vi "HoppingStepModified(XYWithin_And_Nonlinear).vi"() -> ()   [LabVIEW 2014]
uses:
  <vilib>/Platform/TimedLoop/XDataNode/timing_clust.ctl
  <vilib>/Platform/TimedLoop/XDataNode/nitl_modes.ctl
  <vilib>/Platform/TimedLoop/XDataNode/wakeup.ctl
  <vilib>/rvi/Emulation/niFpgaSctlEmulationGetInTimedLoop.vi
  <vilib>/rvi/Emulation/niFpgaProcessEmulError.vi
  <vilib>/rvi/Emulation/niFpgaGetClockAttributes.vi
  <vilib>/rvi/Emulation/niFpgaEmulationReportErrorSimple.vi
  <vilib>/rvi/eio/common/nirviEmuTemplateMethod_errors.vi
  <vilib>/rvi/Emulation/niFpgaCriticalErrorInLSC.vi
  <vilib>/rvi/interface/RandomDataEmulation/niFpgaRandomDataHandleErrors.vi
  <vilib>/eio/EIONode/EIONode.xnode
  <vilib>/Platform/TimedLoop/XDataNode/XDataNode.xnode
  <vilib>/rvi/DataTransferAndStorage/Container/XNode/niFpgaContainer.xnode
  <vilib>/rvi/interface/RandomDataEmulation/nirviRandomDataFpgaReadWriteTemplate.vi
  <vilib>/Platform/TimedLoop/XDataNode/XDNodeRunTimeDep.lvlib
panel:
  out "x >= y?":bool
  out "x*y":i32
  out "CurrDeclineR":i16
  out "ZFreshPos":i16(graph)
  out "Time":i32(graph)
  out "Len":i16(graph)
  out "ZPresPos":i16(graph)
  out "Waveform Chart":i16(graph)
  in  "stop":bool
  in  "MajorWithdraw":i16
  in  "ZOffset":i16
  in  "XNum":i16
  in  "XStepIndex":i16
  in  "XOffset":i16
  in  "YNum":i16
  in  "YStepIndex":i16
  in  "YOffset":i16
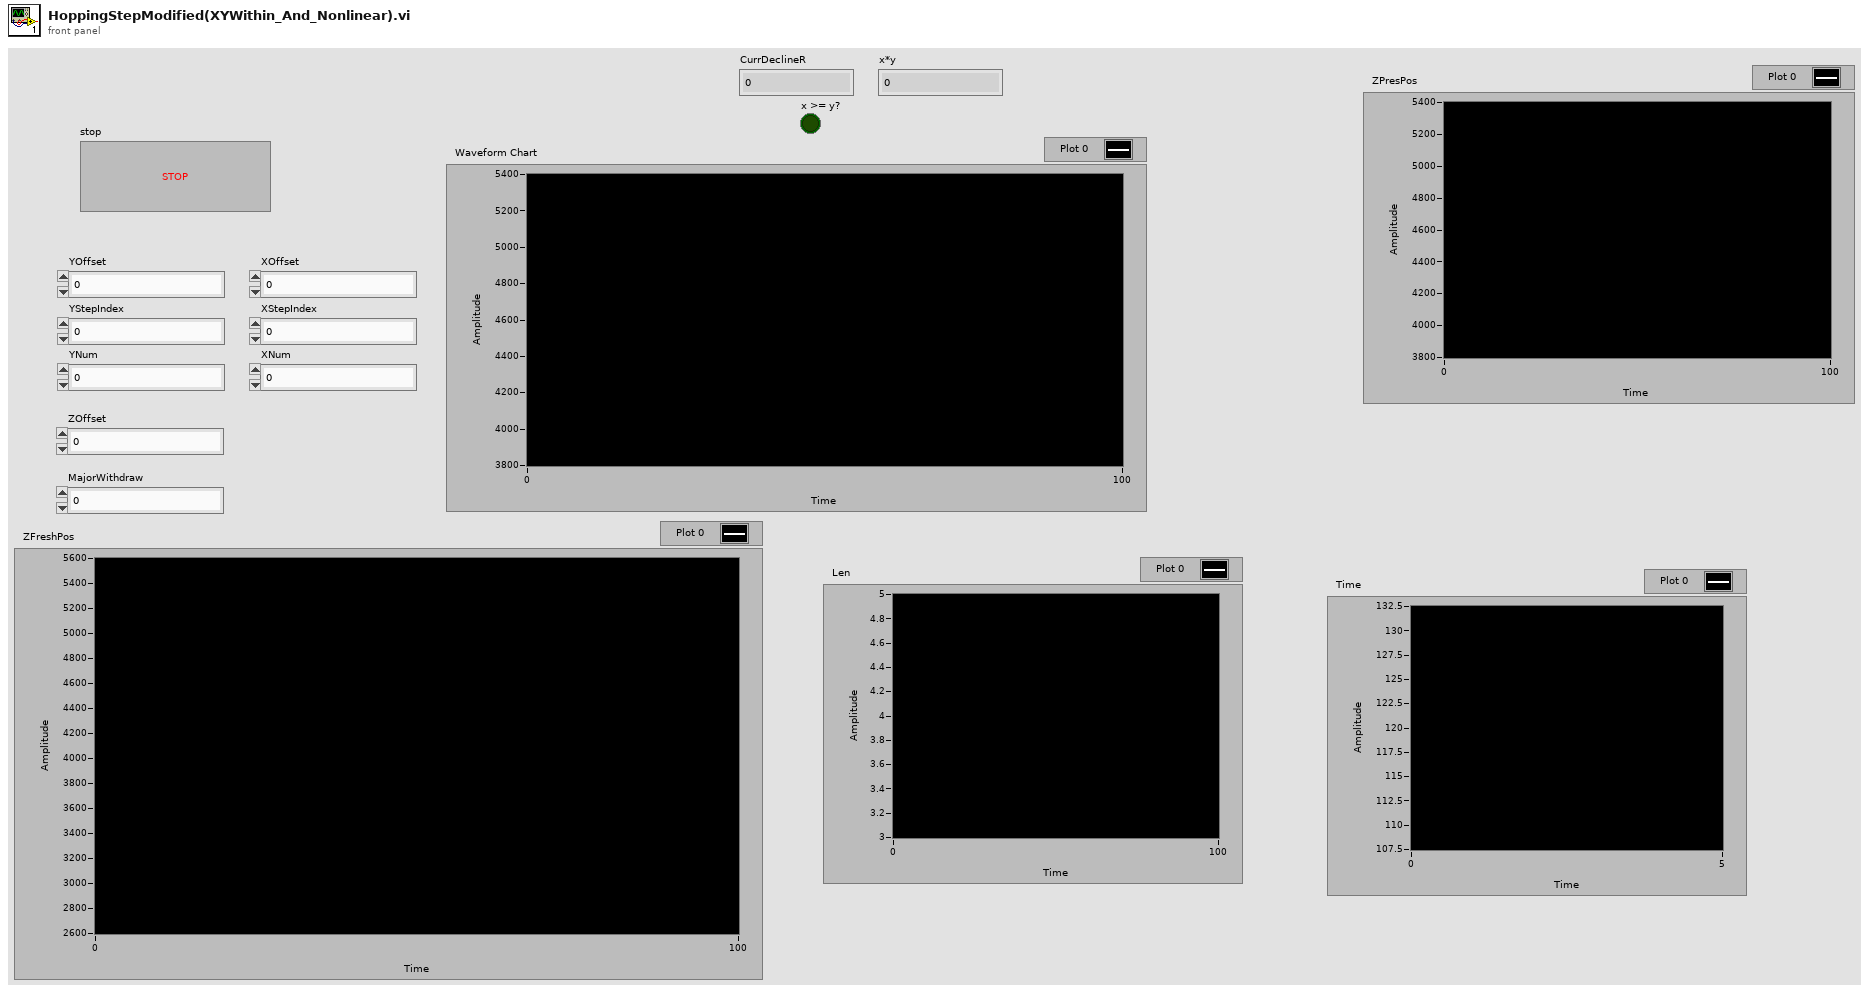
[diagram p1: front panel]
types:
  T1 = typedef "XDNodeRunTimeDep.lvlib/timing_clust.ctl" = cluster{"Expected End [f-1]":u64, "Actual End [f-1]":u64, "Finished Late? [f-1]":bool, "Expected End [i-1]":u64, "Actual End [i-1]":u64, "Finished Late? [i-1]":bool, "Expected Start [i]":u64, "Actual Start [i]":u64, "Expected Start [f]":u64, "Actual Start [f]":u64, "Source Name":string, "Structure Name":string, "Period":i64, "Deadline":i64, "Offset":i64, "Start":i64, "Priority":i32, "Timeout":i32, "Mode":T2, "Wakeup Reason":T3, "Error":errorcluster, "Source Type":string, "Secondary Source Type":string, "Global End Time":u64, "Global Start Time":u64, "Frame Duration":u64, "Iteration Duration":u64, "Assigned CPU":i32, "I/O Scan Engine Mode":u32}
  T2 = typedef "XDNodeRunTimeDep.lvlib/nitl_modes.ctl" = enum32{"No Change", "Process missed periods, maintain original phase", "Discard missed periods, maintain original phase", "Process missed periods, ignore original phase", "Discard missed periods, ignore original phase"}
  T3 = typedef "XDNodeRunTimeDep.lvlib/wakeup.ctl" = enum32{"Normal", "Aborted", "Asynchronous wakeup", "Timing source error", "Timed loop error", "Timeout"}
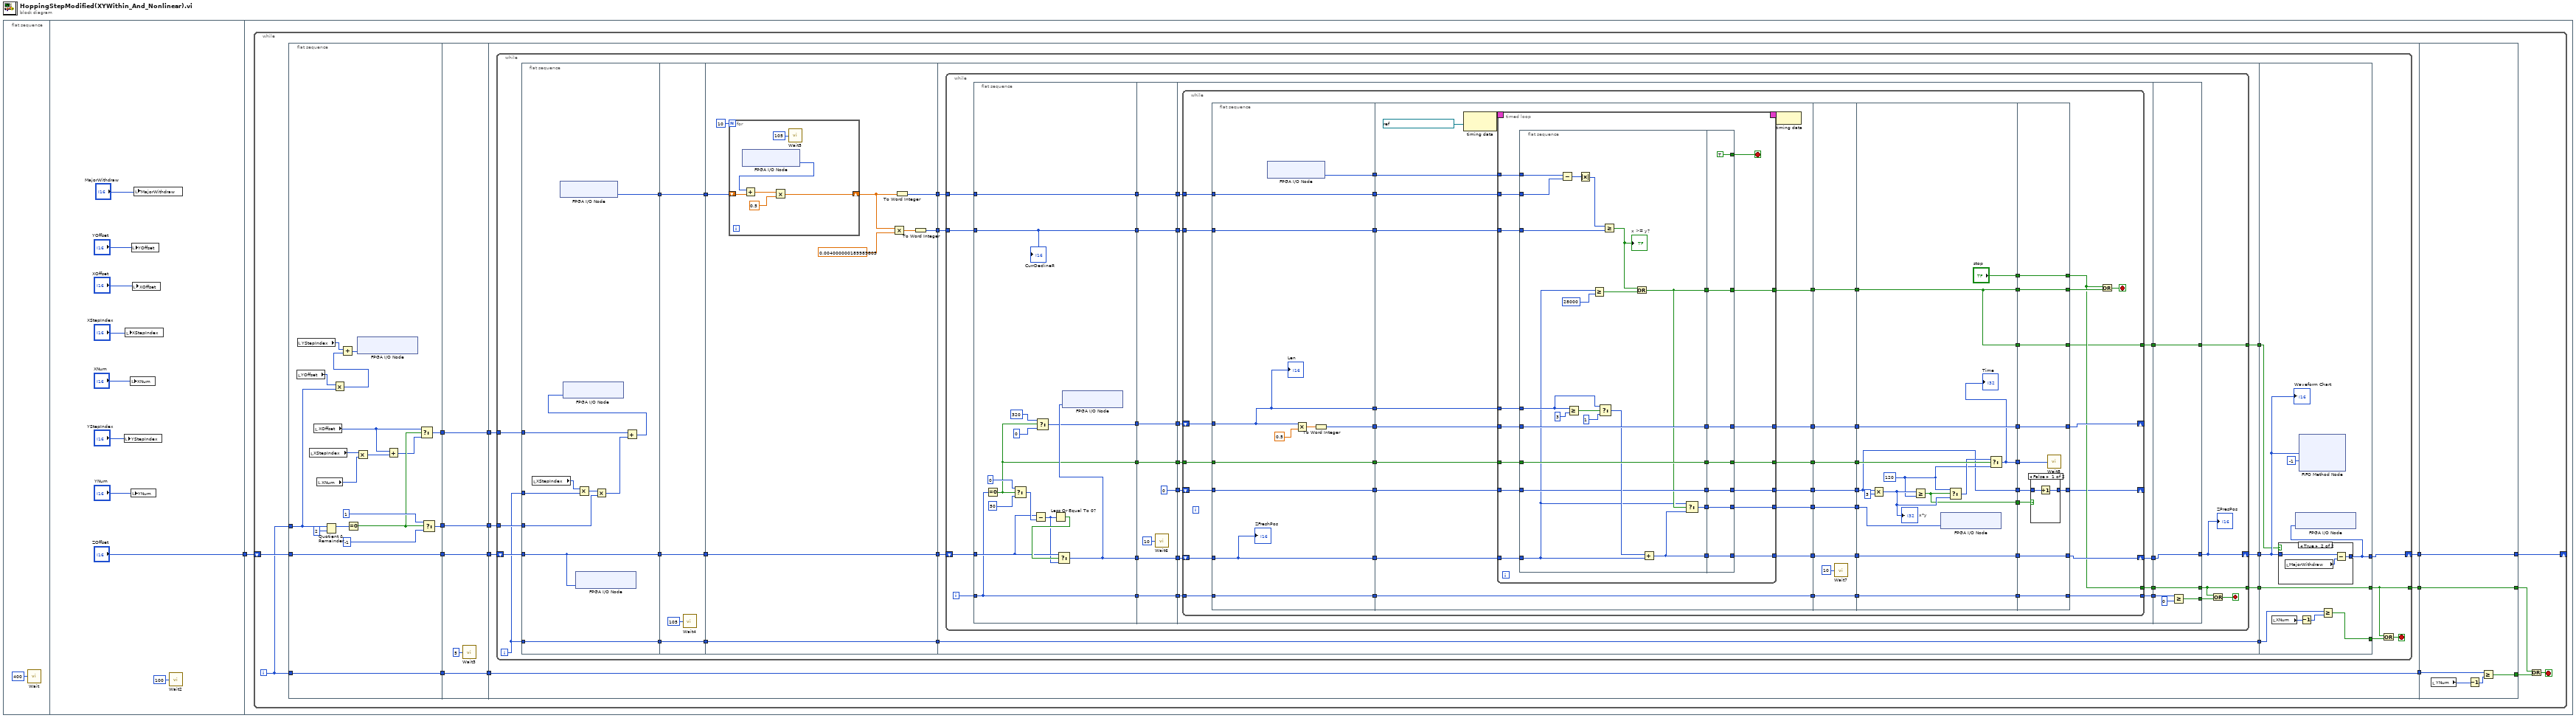
[diagram p0: block diagram]
diagram:
  n1 = flat-sequence {
    tunnel: ["ZOffset"] -> w1
    tunnel: w1 -> [w12]
    frame #0 {
      n2 = call "Wait"("Count(mSec)"=u32 400) -> ()  [unwired: 1 out]
    }
    frame #1 {
      n3 = local write "YStepIndex"("YStepIndex") -> ()
      n4 = local write "XStepIndex"("XStepIndex") -> ()
      n5 = local write "XNum"("XNum") -> ()
      n6 = local write "YNum"("YNum") -> ()
      n7 = local write "YOffset"("YOffset") -> ()
      n8 = local write "XOffset"("XOffset") -> ()
      n9 = local write "MajorWithdraw"("MajorWithdraw") -> ()
      n10 = call "Wait2"("Count(mSec)"=u32 100) -> ()  [unwired: 1 out]
    }
    frame #2 {
      n11 = while {
        shift-right: [w22] -> _
        shift-left: w12 -> [w28]
        i -> [w18]
        stop <- w13 stop-if-true
        n12 = flat-sequence {
          tunnel: w18 -> [w39]
          tunnel: [w44] -> w29
          tunnel: w28 -> [w44]
          tunnel: [w43] -> w25
          tunnel: [w31] -> w23
          tunnel: [w30] -> w19
          tunnel: w18 -> [w30]
          tunnel: w29 -> [w52]
          tunnel: [w52] -> w27
          tunnel: [w51] -> w26
          tunnel: w25 -> [w51]
          tunnel: [w50] -> w24
          tunnel: w23 -> [w50]
          tunnel: w19 -> [w49]
          tunnel: [w49] -> w17
          tunnel: w27 -> [w59]
          tunnel: w26 -> [w58]
          tunnel: w24 -> [w57]
          tunnel: [w56] -> w21
          tunnel: [w55] -> w20
          tunnel: w17 -> [w54]
          tunnel: [w54] -> w16
          tunnel: [w366] -> w22
          tunnel: w21 -> [w366]
          tunnel: w20 -> [w361]
          tunnel: w16 -> [w365]
          tunnel: [w362] -> w15
          tunnel: [w361] -> w14
          frame #0 {
            n13 = local read "YOffset"() -> (w40:i16)
            n14 = local read "YStepIndex"() -> (w42:i16)
            n15 = local read "XStepIndex"() -> (w37:i16)
            n16 = local read "XOffset"() -> (w32:i16)
            n17 = local read "XNum"() -> (w36:i16)
            n18 = Quotient & Remainder(x=w39, y=2) -> (x-y*floor(x/y)=w47:i32)  [unwired: 1 out]
            n19 = Multiply(x=w40, y=w39) -> (x*y=w38:i32)
            n20 = Add(x=w42, y=w38) -> (x+y=w41:i32)
            n21 = Equal To 0?(x=w47) -> (x = 0?=w34:bool)
            n22 = Multiply(x=w37, y=w36) -> (x*y=w35:i16)
            n23 = xnode "FPGA I/O Node"("Connector0/AO3"=w41) -> ()  [unwired: 1 in, 1 out]
            n24 = Add(x=w32, y=w35) -> (x+y=w33:i16)
            n25 = Select(t=w32, s=w34, f=w33) -> (s? t:f=w31:i16)
            n26 = Select(t=1 ("y"), s=w34, f=-1 ("y")) -> (s? t:f=w43:i32)
          }
          frame #1 {
            n27 = call "Wait3"("Count(uSec)"=u32 5) -> ()  [unwired: 1 out]
          }
          frame #2 {
            n28 = while {
              shift-right: [w62] -> w56
              shift-left: w59 -> [w81]
              tunnel: w58 -> [w80]
              tunnel: w57 -> [w79]
              tunnel: [w61] -> w55
              i -> [w67]
              stop <- w70 stop-if-true
              n29 = flat-sequence {
                tunnel: w81 -> [w83]
                tunnel: w80 -> [w88]
                tunnel: w79 -> [w87]
                tunnel: w67 -> [w91]
                tunnel: [w83] -> w77
                tunnel: [w84] -> w75
                tunnel: [w82] -> w68
                tunnel: w67 -> [w82]
                tunnel: [w94] -> w78
                tunnel: w77 -> [w94]
                tunnel: [w93] -> w76
                tunnel: w75 -> [w93]
                tunnel: w68 -> [w92]
                tunnel: [w92] -> w66
                tunnel: w78 -> [w99]
                tunnel: w76 -> [w103]
                tunnel: [w99] -> w74
                tunnel: [w98] -> w73
                tunnel: [w97] -> w72
                tunnel: w66 -> [w96]
                tunnel: [w96] -> w65
                tunnel: w74 -> [w117]
                tunnel: w73 -> [w116]
                tunnel: w72 -> [w115]
                tunnel: [w114] -> w71
                tunnel: [w113] -> w69
                tunnel: w65 -> [w112]
                tunnel: [w112] -> w64
                tunnel: [w111] -> w60
                tunnel: w71 -> [w349]
                tunnel: [w356] -> w62
                tunnel: w69 -> [w355]
                tunnel: [w355] -> w61
                tunnel: w64 -> [w354]
                tunnel: [w351] -> w63
                tunnel: w60 -> [w348]
                frame #0 {
                  n30 = local read "XStepIndex"() -> (w90:i16)
                  n31 = xnode "FPGA I/O Node"() -> ("Connector0/AI1"=w84:i16)  [unwired: 1 in, 1 out]
                  n32 = xnode "FPGA I/O Node"("Connector0/AO0"=w83) -> ()  [unwired: 1 in, 1 out]
                  n33 = Multiply(x=w90, y=w91) -> (x*y=w89:i32)
                  n34 = Multiply(x=w89, y=w88) -> (x*y=w86:i32)
                  n35 = Add(x=w87, y=w86) -> (x+y=w85:i32)
                  n36 = xnode "FPGA I/O Node"("Connector0/AO2"=w85) -> ()  [unwired: 1 in, 1 out]
                }
                frame #1 {
                  n37 = call "Wait4"("Count(uSec)"=u32 105) -> ()  [unwired: 1 out]
                }
                frame #2 {
                  n38 = for {
                    N: 10 -> [_]
                    shift-right: [w105] -> w101
                    shift-left: w103 -> [w109]
                    n39 = xnode "FPGA I/O Node"() -> ("Connector0/AI1"=w108:i16)  [unwired: 1 in, 1 out]
                    n40 = Add(x=w108, y=w109) -> (x+y=w106:sgl)
                    n41 = Multiply(x=w106, y=sgl 0.5) -> (x*y=w105:sgl)
                    n42 = call "Wait5"("Count(uSec)"=u32 105) -> ()  [unwired: 1 out]
                  }
                  n43 = Multiply(x=w101, y=sgl 0.004) -> (x*y=w100:sgl)
                  n44 = To Word Integer(number=w101) -> (16bit integer=w98:i16)
                  n45 = To Word Integer(number=w100) -> (16bit integer=w97:i16)
                }
                frame #3 {
                  n46 = while {
                    shift-right: [w121] -> w114
                    shift-left: w117 -> [w143]
                    tunnel: w116 -> [w142]
                    tunnel: w115 -> [w141]
                    tunnel: [w122] -> w113
                    tunnel: [w118] -> w111
                    i -> [w140]
                    stop <- w125 stop-if-true
                    n47 = flat-sequence {
                      tunnel: w143 -> [w153]
                      tunnel: w142 -> [w150]
                      tunnel: w141 -> [w149]
                      tunnel: w140 -> [w144]
                      tunnel: [w151] -> w138
                      tunnel: [w150] -> w136
                      tunnel: [w149] -> w134
                      tunnel: [w146] -> w132
                      tunnel: [w145] -> w130
                      tunnel: [w144] -> w128
                      tunnel: [w164] -> w139
                      tunnel: w138 -> [w164]
                      tunnel: [w163] -> w137
                      tunnel: w136 -> [w163]
                      tunnel: [w162] -> w135
                      tunnel: w134 -> [w162]
                      tunnel: [w161] -> w133
                      tunnel: w132 -> [w161]
                      tunnel: [w160] -> w131
                      tunnel: w130 -> [w160]
                      tunnel: [w159] -> w129
                      tunnel: w128 -> [w159]
                      tunnel: [i16 0] -> w120
                      tunnel: w139 -> [w176]
                      tunnel: w137 -> [w175]
                      tunnel: w135 -> [w174]
                      tunnel: w133 -> [w173]
                      tunnel: w131 -> [w172]
                      tunnel: w129 -> [w171]
                      tunnel: [w170] -> w127
                      tunnel: [w169] -> w126
                      tunnel: [w168] -> w123
                      tunnel: w120 -> [w167]
                      tunnel: [w166] -> w119
                      tunnel: w127 -> [w347]
                      tunnel: w126 -> [w343]
                      tunnel: [w345] -> w124
                      tunnel: w123 -> [w344]
                      tunnel: [w344] -> w122
                      tunnel: [w343] -> w121
                      tunnel: [w342] -> w118
                      tunnel: w119 -> [w342]
                      frame #0 {
                        n48 = Equal To 0?(x=w144) -> (x = 0?=w145:bool)
                        n49 = Select(t=i16 0, s=w145, f=i16 50) -> (s? t:f=w155:i16)
                        n50 = Subtract(x=w153, y=w155) -> (x-y=w152:i16)
                        n51 = Select(t=i16 320, s=w145, f=i16 0) -> (s? t:f=w146:i16)
                        n52 = Less Or Equal To 0?(x=w152) -> (x <= 0?=w154:bool)
                        n53 = Select(t=w153, s=w154, f=w152) -> (s? t:f=w151:i16)
                        n54 = xnode "FPGA I/O Node"("Connector0/AO0"=w151) -> ()  [unwired: 1 in, 1 out]
                        "CurrDeclineR" <- w149
                      }
                      frame #1 {
                        n55 = call "Wait6"("Count(uSec)"=u32 10) -> ()  [unwired: 1 out]
                      }
                      frame #2 {
                        n56 = while {
                          tunnel: w175 -> [w223]
                          tunnel: w174 -> [w222]
                          shift-right: [w190] -> w169
                          shift-left: w176 -> [w219]
                          shift-right: [w204] -> _
                          shift-left: w173 -> [w221]
                          tunnel: w172 -> [w220]
                          tunnel: w171 -> [w189]
                          tunnel: [w184] -> w170
                          tunnel: [w183] -> w168
                          shift-right: [w180] -> _
                          shift-left: w167 -> [w182]
                          tunnel: [w178] -> w166
                          stop <- w195 stop-if-true
                          n57 = flat-sequence {
                            tunnel: w223 -> [w232]
                            tunnel: w222 -> [w231]
                            tunnel: w221 -> [w226]
                            tunnel: w220 -> [w230]
                            tunnel: w219 -> [w225]
                            tunnel: [w225] -> w218
                            tunnel: [w226] -> w217
                            tunnel: [w232] -> w216
                            tunnel: [w231] -> w215
                            tunnel: [w224] -> w214
                            tunnel: [w230] -> w210
                            tunnel: [w229] -> w207
                            tunnel: [w228] -> w201
                            tunnel: w182 -> [w228]
                            tunnel: w189 -> [w227]
                            tunnel: [w227] -> w188
                            tunnel: w218 -> [w249]
                            tunnel: w217 -> [w248]
                            tunnel: w216 -> [w247]
                            tunnel: w215 -> [w246]
                            tunnel: w214 -> [w245]
                            tunnel: [w244] -> w212
                            tunnel: w210 -> [w243]
                            tunnel: [w242] -> w208
                            tunnel: w207 -> [w241]
                            tunnel: [w240] -> w206
                            tunnel: [w239] -> w202
                            tunnel: w201 -> [w238]
                            tunnel: [w237] -> w200
                            tunnel: [w236] -> w197
                            tunnel: w188 -> [w235]
                            tunnel: [w235] -> w187
                            tunnel: [w314] -> w213
                            tunnel: w212 -> [w314]
                            tunnel: [w313] -> w209
                            tunnel: w208 -> [w313]
                            tunnel: w206 -> [w312]
                            tunnel: [w312] -> w205
                            tunnel: [w310] -> w203
                            tunnel: w202 -> [w310]
                            tunnel: w200 -> [w307]
                            tunnel: [w307] -> w199
                            tunnel: w197 -> [w309]
                            tunnel: [w309] -> w196
                            tunnel: w187 -> [w308]
                            tunnel: [w308] -> w186
                            tunnel: w213 -> [w328]
                            tunnel: [w328] -> w211
                            tunnel: w209 -> [w326]
                            tunnel: w205 -> [w327]
                            tunnel: w203 -> [w320]
                            tunnel: w199 -> [w317]
                            tunnel: [w318] -> w198
                            tunnel: w196 -> [w315]
                            tunnel: [w315] -> w194
                            tunnel: ["stop"] -> w192
                            tunnel: [w320] -> w191
                            tunnel: w186 -> [w319]
                            tunnel: [w319] -> w185
                            tunnel: [w317] -> w181
                            tunnel: [w316] -> w179
                            tunnel: [w315] -> w177
                            tunnel: w211 -> [w338]
                            tunnel: [w338] -> w204
                            tunnel: w198 -> [w329]
                            tunnel: [w337] -> w193
                            tunnel: w194 -> [w337]
                            tunnel: [w336] -> w183
                            tunnel: w192 -> [w336]
                            tunnel: [w335] -> w190
                            tunnel: w191 -> [w335]
                            tunnel: w185 -> [w334]
                            tunnel: [w334] -> w184
                            tunnel: w181 -> [w332]
                            tunnel: [w331] -> w180
                            tunnel: w179 -> [w333]
                            tunnel: [w330] -> w178
                            tunnel: w177 -> [w330]
                            frame #0 {
                              n58 = xnode "FPGA I/O Node"() -> ("Connector0/AI1"=w229:i16)  [unwired: 1 in, 1 out]
                              n59 = Multiply(x=w226, y=sgl 0.5) -> (x*y=w233:sgl)
                              n60 = To Word Integer(number=w233) -> (16bit integer=w224:i16)
                              "Len" <- w226
                              "ZFreshPos" <- w225
                            }
                            frame #1 {
                              n61 = node-c288(refnum<k21> "40 MHz Onboard Clock" ("Source Name")) -> (w252:T1)
                              n62 = timed-loop {
                                timing: w252 -> [_]
                                timing-out: [_] -> w251
                                tunnel: w249 -> [w268]
                                tunnel: w248 -> [w273]
                                tunnel: [w269] -> w239
                                tunnel: w247 -> [w271]
                                tunnel: w246 -> [w270]
                                tunnel: w245 -> [w266]
                                tunnel: [w265] -> w244
                                tunnel: w243 -> [w264]
                                tunnel: [w263] -> w242
                                tunnel: w241 -> [w272]
                                tunnel: [w267] -> w240
                                tunnel: w238 -> [w256]
                                tunnel: [w255] -> w237
                                tunnel: [w254] -> w236
                                stop <- w258 stop-if-true
                                n63 = flat-sequence {
                                tunnel: w273 -> [w279]
                                tunnel: w272 -> [w293]
                                tunnel: w271 -> [w292]
                                tunnel: w270 -> [w290]
                                tunnel: w268 -> [w275]
                                tunnel: w266 -> [w284]
                                tunnel: w264 -> [w283]
                                tunnel: [w274] -> w262
                                tunnel: [w285] -> w261
                                tunnel: [w284] -> w260
                                tunnel: [w283] -> w259
                                tunnel: [w277] -> w257
                                tunnel: w256 -> [w277]
                                tunnel: [w276] -> w253
                                tunnel: [w297] -> w263
                                tunnel: [w298] -> w265
                                tunnel: [w299] -> w267
                                tunnel: [w300] -> w269
                                tunnel: w262 -> [w300]
                                tunnel: w261 -> [w299]
                                tunnel: w260 -> [w298]
                                tunnel: w259 -> [w297]
                                tunnel: [TRUE] -> w258
                                tunnel: [w295] -> w255
                                tunnel: w257 -> [w295]
                                tunnel: [w294] -> w254
                                tunnel: w253 -> [w294]
                                frame #0 {
                                n64 = Subtract(x=w293, y=w292) -> (x-y=w291:i16)
                                n65 = Greater Or Equal?(x=w279, y=i16 3) -> (x >= y?=w281:bool)
                                n66 = Absolute Value(x=w291) -> (abs(x)=w289:i16)
                                n67 = Greater Or Equal?(x=w275, y=i16 28000) -> (x >= y?=w287:bool)
                                n68 = Select(t=w279, s=w281, f=i16 1 ("y")) -> (s? t:f=w278:i16)
                                n69 = Greater Or Equal?(x=w289, y=w290) -> (x >= y?=w288:bool)
                                "x >= y?" <- w288
                                n70 = Or(x=w288, y=w287) -> (x .or. y?=w276:bool)
                                n71 = Add(x=w278, y=w275) -> (x+y=w274:i16)
                                n72 = Select(t=w275, s=w276, f=w274) -> (s? t:f=w285:i16)
                                }
                                frame #1 {
                                }
                                }
                              }
                              n73 = node-c288(w251) -> ()
                            }
                            frame #2 {
                              n74 = call "Wait7"("Count(uSec)"=u32 10) -> ()  [unwired: 1 out]
                            }
                            frame #3 {
                              w322 = 120 ("y")
                              n75 = Multiply(x=w317, y=3) -> (x*y=w324:i32)
                              "x*y" <- w324
                              n76 = Greater Or Equal?(x=w324, y=w322) -> (x >= y?=w316:bool)
                              n77 = xnode "FPGA I/O Node"("Connector0/AO0"=w327) -> ()  [unwired: 1 in, 1 out]
                              n78 = Select(t=w322, s=w316, f=w324) -> (s? t:f=w323:i32)
                              n79 = Select(t=w323, s=w326, f=w322) -> (s? t:f=w318:i32)
                              "Time" <- w318
                            }
                            frame #4 {
                              n80 = case shown="False" w333 {
                                tunnel: w332 -> [w340 w341]
                                tunnel: [w339 w341] -> w331
                                frame False {
                                n81 = Increment(x=w340) -> (x+1=w339:i16)
                                }
                                frame True {
                                }
                              }
                              n82 = call "Wait8"("Count(uSec)"=w329) -> ()  [unwired: 1 out]
                            }
                          }
                          n83 = Or(x=w183, y=w193) -> (x .or. y?=w195:bool)
                        }
                      }
                      frame #3 {
                        n84 = Greater Or Equal?(x=w347, y=0) -> (x >= y?=w345:bool)
                      }
                    }
                    n85 = Or(x=w122, y=w124) -> (x .or. y?=w125:bool)
                    "ZPresPos" <- w121
                  }
                }
                frame #4 {
                  n86 = local read "XNum"() -> (w353:i16)
                  n87 = case shown="True" w348 {
                    tunnel: [w357 w359] -> w356
                    tunnel: w349 -> [w357 w358]
                    frame False {
                    }
                    frame True {
                      n88 = local read "MajorWithdraw"() -> (w360:i16)
                      n89 = Subtract(x=w358, y=w360) -> (x-y=w359:i16)
                    }
                  }
                  n90 = xnode "FPGA I/O Node"("Connector0/AO0"=w356) -> ()  [unwired: 1 in, 1 out]
                  n91 = xnode ("FIFO Method Node")("Element"=w349, "Timeout"=-1) -> ()  [unwired: 1 in, 2 out]
                  n92 = Decrement(x=w353) -> (x-1=w352:i16)
                  n93 = Greater Or Equal?(x=w354, y=w352) -> (x >= y?=w351:bool)
                  "Waveform Chart" <- w349
                }
              }
              n94 = Or(x=w61, y=w63) -> (x .or. y?=w70:bool)
            }
          }
          frame #3 {
            n95 = local read "YNum"() -> (w363:i16)
            n96 = Decrement(x=w363) -> (x-1=w364:i16)
            n97 = Greater Or Equal?(x=w365, y=w364) -> (x >= y?=w362:bool)
          }
        }
        n98 = Or(x=w14, y=w15) -> (x .or. y?=w13:bool)
      }
    }
  }
